vi "WSVCAP SHL Host TL Tester.vi"() -> ()   [LabVIEW 2012]
uses:
  Type Defs/WSVCAP SHL DUT Number Enum.ctl
  <vilib>/userdefined/High Color/nirio_resource_hc.ctl
  Type Defs/WSVCAP SHL Tester System Cluster.ctl
  Type Defs/WSVCAP SHL I2C DUT Mask Mode Enum.ctl
panel:
  in  "C3 Cap DAC":u8=144 caption="B Data In" format="0x%02x"
  in  "C2 Cap DAC":u8=144 caption="B Data In" format="0x%02x"
  in  "C1 Cap DAC":u8=144 caption="B Data In" format="0x%02x"
  in  "Set Cap DAC":bool
  in  "CP 35V":bool
  in  "CP 23.75V":bool
  in  "DVA On":bool
  in  "DVA Off":bool
  in  "CP 44V":bool
  in  "CP 40.25V":bool
  in  "Read Data DUT CMD":string caption="Read Data Out"
  in  "Read DUT":bool
  in  "CP On":bool
  in  "CP Off":bool
  in  "Write DUT":bool
  in  "Write Data DUT":string caption="Write Data Out"
  out "Read Data DUT Out":string caption="Data In"
  in  "Stop RFFE Cycle":bool
  in  "Start RFFE Cycle":bool
  in  "Command":string[](array[string])=["702013B3B3B", "70201000000"]
  in  "Post CMd Delay":dbl[](array[numeric])=[1.2e-05, 5.4e-05] min=0.0 max=0.5 format="%#.0p s"
  in  "Number of Commands":u32=2 min=1 max=4 step=1
  out "Cycle Count":u64=2 min=1 max=4 step=1
  in  "Monitor":bool
  out "AD7747 Values":string[][](table)
  in  "Mode":enum32{"C1", "C2", "C3", "All", "Single"}(radio)
  in  "RFFE Slave Address":u8=144 caption="Slave Address" format="0x%02x"
  out "Activity Log":string
  out "Simulate FPGA":bool
  out "Online":bool
  out "FPGA Resource":T1
  out "Status":string
  out "Busy":bool
  in  "I2C Bytes to Read":u8=1 caption="Bytes" min=1 max=4 step=1
  in  "Device":enum32{"C1", "C2", "C3"}(radio)
  in  "Exit":bool
  out "Read Data I2C":u8[](array[numeric]) caption="Data In" format="0x%02x"
  in  "Read Reg I2C":u8 caption="Register" format="0x%02x"
  in  "Read I2C":bool
  in  "DUT":T2
  in  "Write Data I2C":u8 caption="Data Out" format="0x%02x"
  in  "Write Reg I2C":u8=144 caption="Register" format="0x%02x"
  in  "I2C Init":bool
  in  "Init Data":u8[](array[numeric])=[164, 160, 14, 33] caption="Data Out" format="0x%02x"
  in  "Init Reg":u8[](array[numeric])=[191, 7, 9, 10] caption="Register" format="0x%02x"
  in  "Write I2C":bool
  in  "I2C Slave Address":u8=144 caption="Slave Address" format="0x%02x"
  in  "RFFE Clock Rate (Hz)":dbl=1000000.0 caption="Clock Rate" format="%.1p Hz"
  in  "I2C Clock Rate (Hz)":dbl=100000.0 caption="Clock Rate" format="%.0p Hz"
  in  "Error":errorcluster
  # "WS1050 Tester"
  # "AD7747 (I2C)"
  # "C1"
  # "C2"
  # "C3"
  # "DUT Control (RFFE)"
  # "DUT Cycling (RFFE)"
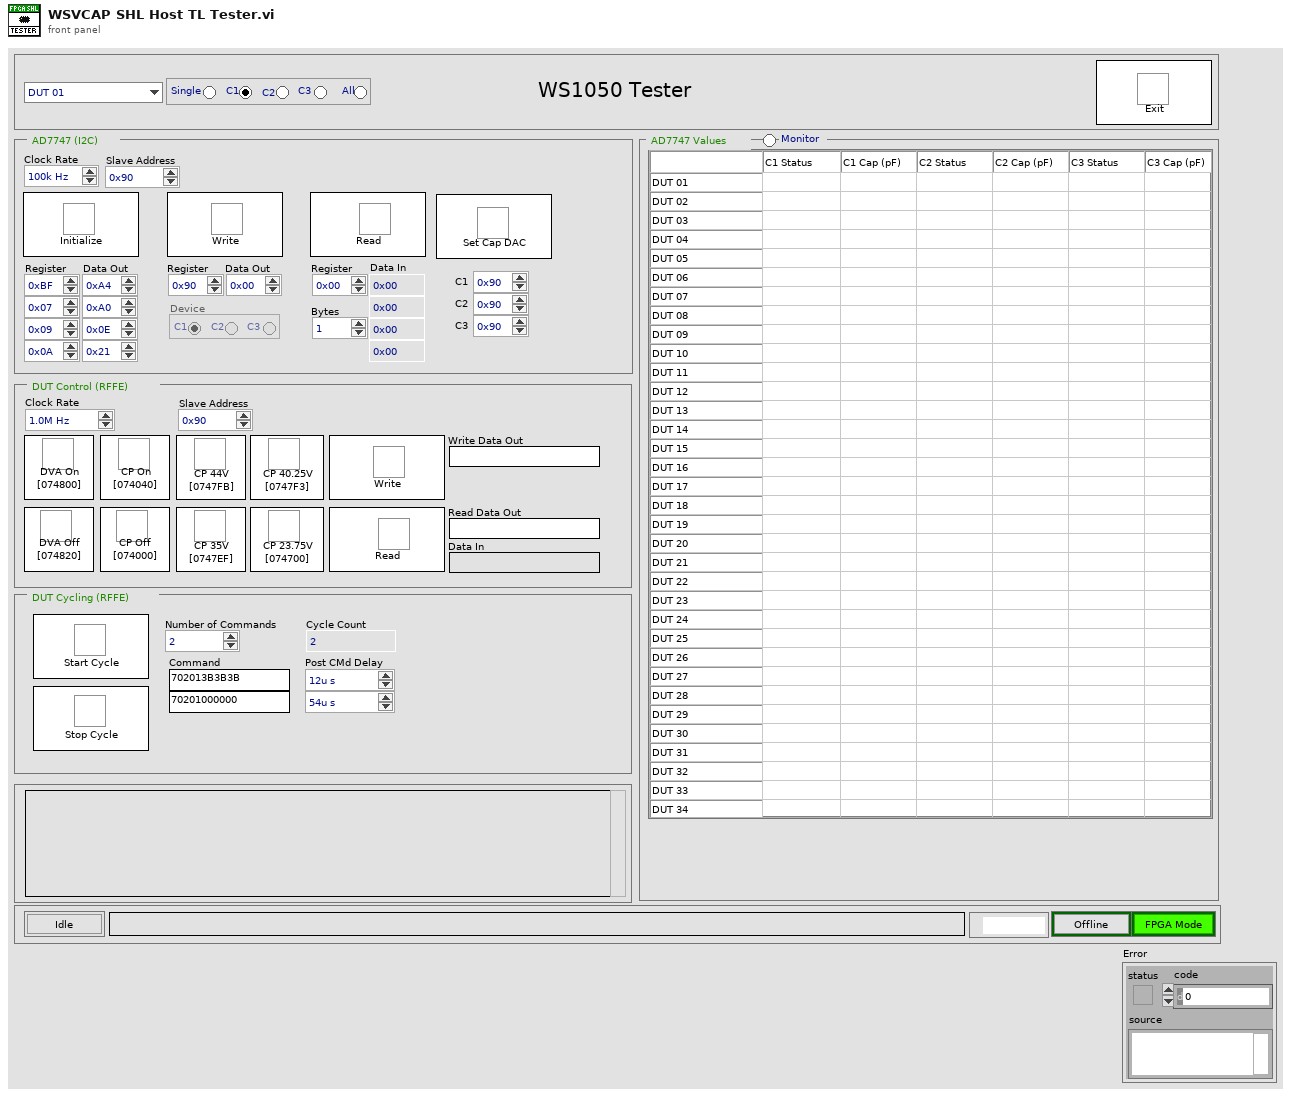
[diagram p1: front panel]
types:
  T1 = typedef "nirio_resource_hc.ctl" = tag
  T2 = typedef "WSVCAP SHL DUT Number Enum.ctl" = enum16{"DUT 01", "DUT 02", "DUT 03", "DUT 04", "DUT 05", "DUT 06", "DUT 07", "DUT 08", "DUT 09", "DUT 10", "DUT 11", "DUT 12", "DUT 13", "DUT 14", "DUT 15", "DUT 16", "DUT 17", "DUT 18", "DUT 19", "DUT 20", "DUT 21", "DUT 22", "DUT 23", "DUT 24", "DUT 25", "DUT 26", "DUT 27", "DUT 28", "DUT 29", "DUT 30", "DUT 31", "DUT 32", "DUT 33", "DUT 34", "DUT 35", "DUT 36"}
  T3 = typedef "WSVCAP SHL Tester System Cluster.ctl" = cluster{"I2C Monitor":bool, "SPI Cyle":bool, "SPI Mode":enum32{"Write/Read", "Cycle"}, "RFFE Cyle":bool, "RFFE Mode":enum32{"Write/Read", "Cycle"}}
  T4 = typedef "WSVCAP SHL Core System Cluster.ctl" = cluster{"Settings":T5, "FPGA Resource":tag, "Online":bool, "I2C Wait Ticks":u32, "SPI Wait Ticks":u32, "RFFE Wait Ticks":u32}
  T5 = typedef "WSVCAP SHL I2C Settings Cluster.ctl" = cluster{"FPGA Resource Name":string, "I2C Slave Address":u8, "I2C Clock Rate (Hz)":dbl, "SPI Clock Rate (Hz)":dbl, "RFFE Slave Address":u8, "RFFE Clock Rate (Hz)":dbl, "Simulate FPGA":bool, "C1 Cap DAC Default":u8, "C2 Cap DAC Default":u8, "C3 Cap DAC Default":u8}
  T6 = enum8{"Enabled", "Disabled", "Disabled and Grayed Out"}
  T7 = typedef "WSVCAP SHL I2C DUT Mask Mode Enum.ctl" = enum16{"Custom", "C1", "C2", "C3", "All"}
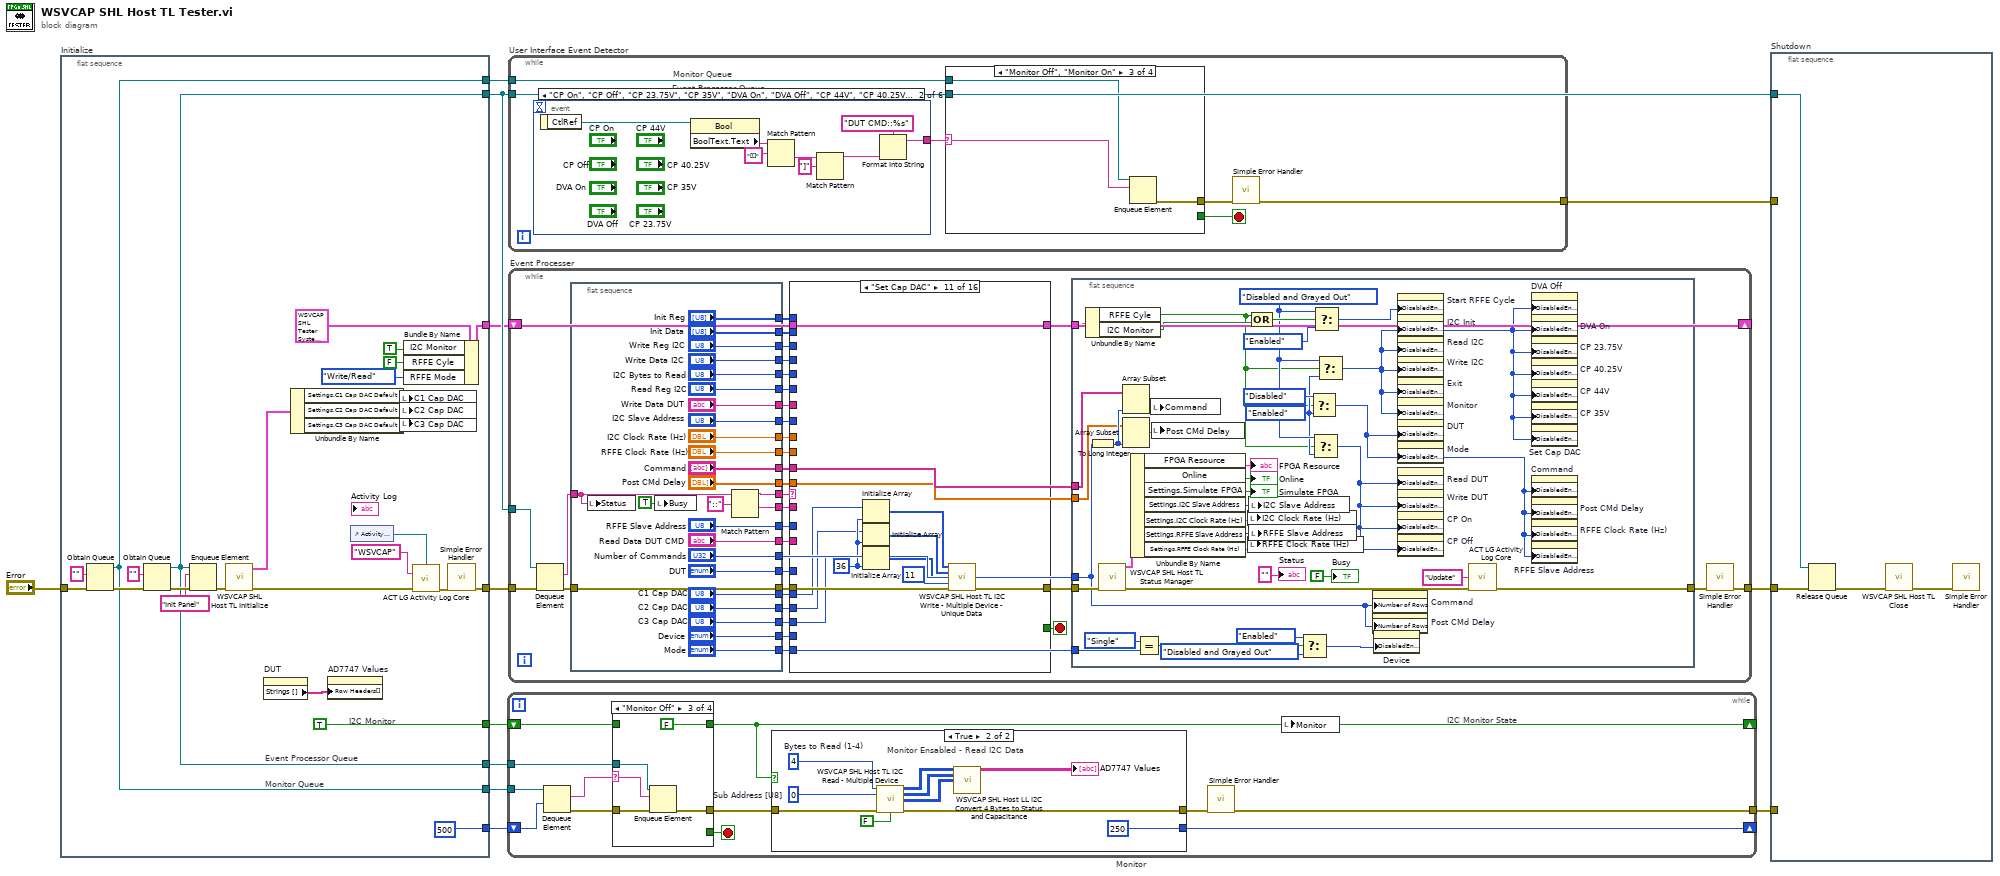
[diagram p0: block diagram]
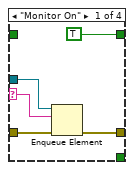
[diagram p2: hidden frame]
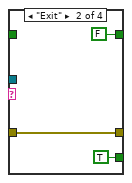
[diagram p3: hidden frame]
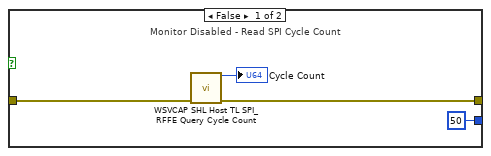
[diagram p5: hidden frame]
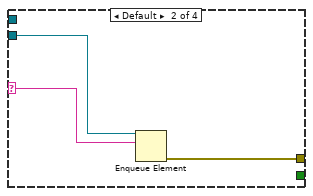
[diagram p7: hidden frame]
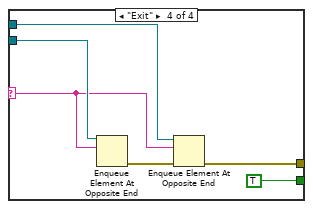
[diagram p8: hidden frame]
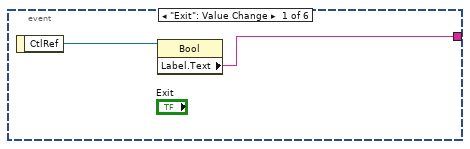
[diagram p9: hidden frame]
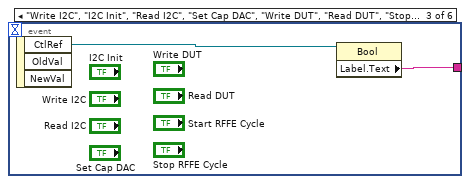
[diagram p10: hidden frame]
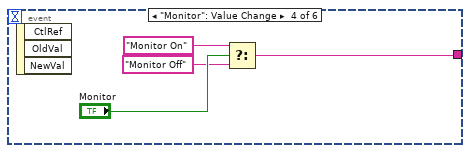
[diagram p11: hidden frame]
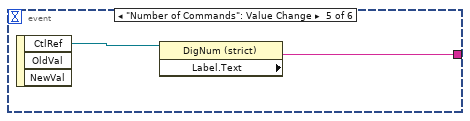
[diagram p12: hidden frame]
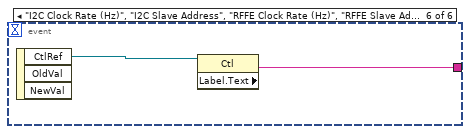
[diagram p13: hidden frame]
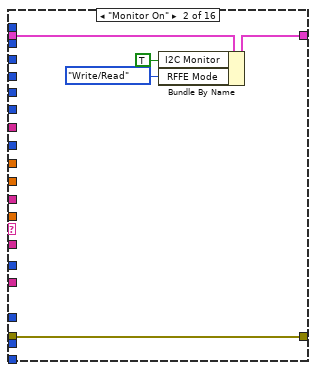
[diagram p15: hidden frame]
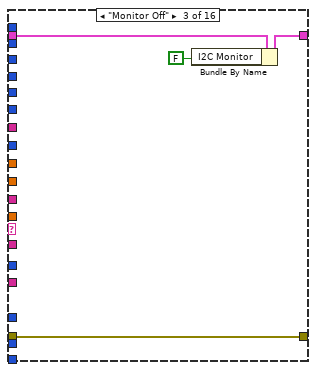
[diagram p16: hidden frame]
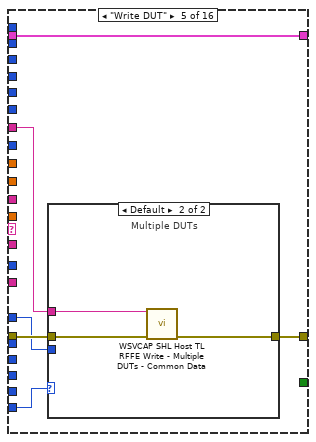
[diagram p18: hidden frame]
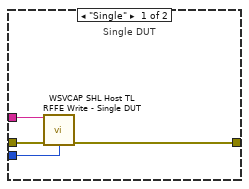
[diagram p19: hidden frame]
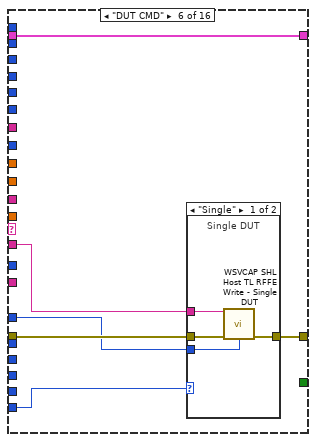
[diagram p20: hidden frame]
diagram:
  n1 = flat-sequence "Initialize" {
    tunnel: "Error" -> [w29]
    tunnel: [w27] -> w11
    tunnel: [TRUE ("Monitor")] -> w2
    tunnel: [w34] -> w7
    tunnel: [w25] -> w6
    tunnel: [w22] -> w5
    tunnel: [w27] -> w4
    tunnel: [w22] -> w3
    tunnel: [500 ("Wait Time (500ms)")] -> w1
    frame #0 {
      # "I2C Monitor"
      # "Monitor Queue"
      # "Event Processor Queue"
      n2 = Obtain Queue(element data type="" ("name (unnamed)"), error in (no error)=w29) -> (queue out=w22:refnum<queue>, error out=w28:errorcluster)  [unwired: 3 in, 1 out]
      n3 = Obtain Queue(element data type="" ("name (unnamed)"), error in (no error)=w28) -> (queue out=w27:refnum<queue>, error out=w37:errorcluster)  [unwired: 3 in, 1 out]
      n4 = Enqueue Element(queue=w27, element="Init Panel" ("name (unnamed)"), error in (no error)=w37) -> (error out=w19:errorcluster)  [unwired: 1 in, 2 out]
      n5 = call "WSVCAP SHL Host TL Initialize.vi"("error in"=w19) -> ("System"=w17:T4, "error out"=w18:errorcluster)  [unwired: 13 in]
      n6 = property on="DUT" class="Enum (strict)"() -> ("Strings []"=w20:string[])  [unwired: 2 in, 2 out]
      n7 = Unbundle By Name(w17) -> ("Settings.C1 Cap DAC Default"=w16:u8, "Settings.C2 Cap DAC Default"=w15:u8, "Settings.C3 Cap DAC Default"=w14:u8)
      n8 = property on="AD7747 Values" class="Tbl (strict)"("Row Headers[]"=w20) -> ()  [unwired: 2 in, 2 out]
      n9 = control-ref of="Activity Log"() -> (w33:refnum<vi>)
      n10 = local write "C1 Cap DAC"(w16) -> ()
      n11 = local write "C2 Cap DAC"(w15) -> ()
      n12 = local write "C3 Cap DAC"(w14) -> ()
      n13 = Bundle By Name(cluster=T3 {"I2C Monitor"=TRUE, "SPI Cyle"=TRUE, "SPI Mode"=enum."Write/Read", "RFFE Cyle"=FALSE, "RFFE Mode"=enum."Write/Read"}, "I2C Monitor"=TRUE, "RFFE Cyle"=FALSE ("I2C Monitor"), "RFFE Mode"=enum32{"Write/Read", "Cycle"}."Write/Read" ("SPI Mode")) -> (w25:T3)
      n14 = call "ACT LG Activity Log Core.vi"("Display Ref"=w33, "Source"="WSVCAP", "Error In (no error)"=w18) -> ("Error Out"=w35:errorcluster)  [unwired: 11 in, 1 out]
      n15 = call <vilib>:"Simple Error Handler.vi"("error in (no error)"=w35) -> ("error out"=w34:errorcluster)  [unwired: 4 in, 4 out]
    }
  }
  n16 = while "Monitor" {
    tunnel: [w42] -> w8
    shift-right: [w41] -> _
    shift-left: w2 -> [w48]
    tunnel: w5 -> [w46]
    tunnel: w4 -> [w45]
    shift-right: [w40] -> _
    shift-left: w1 -> [w39]
    stop <- w43 stop-if-true
    # "I2C Monitor State"
    n17 = Dequeue Element(queue=w46, timeout in ms (-1)=w39) -> (element=w49:string, error out=w47:errorcluster)  [unwired: 1 in, 2 out]
    n18 = case shown="\"Monitor Off\"" w49 {
      selector: w49 -> [w52 _ w60 _]
      tunnel: [TRUE FALSE FALSE w65] -> w41
      tunnel: w48 -> [_ _ _ w65]
      tunnel: w47 -> [w54 w57 w62 w64]
      tunnel: [w53 w57 w61 w64] -> w44
      tunnel: w45 -> [w51 _ w59 _]
      tunnel: [_ TRUE _ _] -> w43
      frame "Monitor On" {
        n19 = Enqueue Element(queue=w51, element=w52, error in (no error)=w54) -> (error out=w53:errorcluster)  [unwired: 1 in, 2 out]
      }
      frame "Exit" {
      }
      frame "Monitor Off" {
        n20 = Enqueue Element(queue=w59, element=w60, error in (no error)=w62) -> (error out=w61:errorcluster)  [unwired: 1 in, 2 out]
      }
      frame Default {
      }
    }
    n21 = case shown="True" w41 {
      tunnel: [w67 w73] -> w50
      tunnel: w44 -> [w68 w74]
      tunnel: [50 ("Wait Time (500ms)") 250 ("Wait Time (500ms)")] -> w40
      frame False {
        # "Monitor Disabled - Read SPI Cycle Count"
        n22 = call "WSVCAP SHL Host TL SPI_RFFE Query Cycle Count.vi"("error in"=w68) -> ("Cycle Count"=→"Cycle Count":u64, "error out"=w67:errorcluster)  [unwired: 13 in]
      }
      frame True {
        w78 = u8 4  # Bytes to Read (1-4)
        w79 = u8 0  # Sub Address [U8]
        # "Monitor Ensabled - Read I2C Data"
        n23 = call "WSVCAP SHL Host TL I2C Read - Multiple Device.vi"("Bytes to Read (1-4)"=w78, "Sub Address [U8]"=w79, "error in"=w74, "Log (T)"=FALSE) -> ("C1:1-36 Read Data [U8]"=w77:u8[][], "C2:1-36 Read Data [U8]"=w76:u8[][], "C3:1-36 Read Data [U8]"=w72:u8[][], "error out"=w73:errorcluster)  [unwired: 8 in]
        n24 = call "WSVCAP SHL Host LL I2C Convert 4 Bytes to Status and Capacitance.vi"("C1:1-36 Read Data [U8]"=w77, "C2_1-36 Read Data [U8]"=w76, "C3_1-36 Read Data [U8]"=w72) -> ("AD7747 Values"=→"AD7747 Values":string[][])  [unwired: 12 in]
      }
    }
    n25 = call <vilib>:"Simple Error Handler.vi"("error in (no error)"=w50) -> ("error out"=w42:errorcluster)  [unwired: 4 in, 4 out]
    n26 = local write "Monitor"(w41) -> ()
  }
  n27 = while "User Interface Event Detector" {
    tunnel: w11 -> [w84]
    tunnel: [w81] -> w9
    tunnel: w3 -> [w80]
    stop <- w82 stop-if-true
    # "Monitor Queue"
    # "Event Processor Queue"
    n28 = event shown="[1] \"CP On\", \"CP Off\", \"CP 23.75V\", \"CP 35V\", \"DVA On\", \"DVA Off\", \"CP 44V\", \"CP 40.25V\": Value Change" {
      selector: _ -> [_ _ _ _ _ _]
      dyn-events: _ -> [_ _ _ _ _ _]
      timeout: _ -> [_ _ _ _ _ _]
      tunnel: [w98 w106 w109 w110 w115 w117] -> w85
      event "Exit": Value Change {
        n29 = event-data() -> ("CtlRef"=w99:refnum<vi>)  [unwired: 1 in]
        n30 = property class="Bool"(reference=w99) -> ("Label.Text"=w98:string)  [unwired: 1 in, 2 out]
      }
      event "CP On", "CP Off", "CP 23.75V", "CP 35V", "DVA On", "DVA Off", "CP 44V", "CP 40.25V": Value Change {
        n31 = event-data() -> ("CtlRef"=w107:refnum<vi>)  [unwired: 1 in]
        n32 = property class="Bool"(reference=w107) -> ("BoolText.Text"=w104:string)  [unwired: 1 in, 2 out]
        n33 = Match Pattern(string=w104, regular expression="[[]") -> (after substring=w102:string)  [unwired: 1 in, 3 out]
        n34 = Match Pattern(string=w102, regular expression="]") -> (before substring=w100:string)  [unwired: 1 in, 3 out]
        n35 = Format Into String(format string="DUT CMD::%s", w100) -> (resulting string=w106:string)  [unwired: 2 in, 1 out]
      }
      event "Write I2C", "I2C Init", "Read I2C", "Set Cap DAC", "Write DUT", "Read DUT", "Stop RFFE Cycle", "Start RFFE Cycle": Value Change {
        n36 = event-data() -> ("CtlRef"=w108:refnum<vi>)  [unwired: 1 in, 2 out]
        n37 = property class="Bool"(reference=w108) -> ("Label.Text"=w109:string)  [unwired: 1 in, 2 out]
      }
      event "Monitor": Value Change {
        n38 = event-data() -> ()  [unwired: 1 in, 3 out]
        n39 = Select(t="Monitor On" ("Label.Text"), s="Monitor", f="Monitor Off" ("Label.Text")) -> (s? t:f=w110:string)
      }
      event "Number of Commands": Value Change {
        n40 = event-data() -> ("CtlRef"=w114:refnum<vi>)  [unwired: 1 in, 2 out]
        n41 = property class="DigNum (strict)"(reference=w114) -> ("Label.Text"=w115:string)  [unwired: 1 in, 2 out]
      }
      event "I2C Clock Rate (Hz)", "I2C Slave Address", "RFFE Clock Rate (Hz)", "RFFE Slave Address", "Mode": Value Change {
        n42 = event-data() -> ("CtlRef"=w116:refnum<vi>)  [unwired: 1 in, 2 out]
        n43 = property class="Ctl"(reference=w116) -> ("Label.Text"=w117:string)  [unwired: 1 in, 2 out]
      }
    }
    n44 = case shown="\"Monitor Off\", \"Monitor On\"" w85 {
      selector: w85 -> [_ w88 w91 w92]
      tunnel: w84 -> [_ w87 _ w97]
      tunnel: [_ w86 w90 w94] -> w83
      tunnel: [_ _ _ TRUE] -> w82
      tunnel: w80 -> [_ _ w89 w93]
      frame "" {
      }
      frame Default {
        n45 = Enqueue Element(queue=w87, element=w88) -> (error out=w86:errorcluster)  [unwired: 2 in, 2 out]
      }
      frame "Monitor Off", "Monitor On" {
        n46 = Enqueue Element(queue=w89, element=w91) -> (error out=w90:errorcluster)  [unwired: 2 in, 2 out]
      }
      frame "Exit" {
        n47 = Enqueue Element At Opposite End(queue=w97, element=w92) -> (error out=w95:errorcluster)  [unwired: 2 in, 2 out]
        n48 = Enqueue Element At Opposite End(queue=w93, element=w92, error in (no error)=w95) -> (error out=w94:errorcluster)  [unwired: 1 in, 2 out]
      }
    }
    n49 = call <vilib>:"Simple Error Handler.vi"("error in (no error)"=w83) -> ("error out"=w81:errorcluster)  [unwired: 4 in, 4 out]
  }
  n50 = while "Event Processer" {
    tunnel: w11 -> [w151]
    tunnel: [w149] -> w10
    tunnel: w7 -> [w130]
    shift-right: [w125] -> _
    shift-left: w6 -> [w126]
    stop <- w150 stop-if-true
    n51 = Dequeue Element(queue=w151, error in (no error)=w130) -> (element=w147:string, error out=w145:errorcluster)  [unwired: 1 in, 2 out]
    n52 = flat-sequence {
      tunnel: ["I2C Clock Rate (Hz)"] -> w148
      tunnel: [w195] -> w146
      tunnel: w147 -> [w196]
      tunnel: [w215] -> w144
      tunnel: w145 -> [w215]
      tunnel: ["I2C Bytes to Read"] -> w143
      tunnel: ["I2C Slave Address"] -> w142
      tunnel: ["RFFE Clock Rate (Hz)"] -> w141
      tunnel: ["DUT"] -> w138
      tunnel: ["Init Data"] -> w137
      tunnel: ["Init Reg"] -> w136
      tunnel: ["Write Reg I2C"] -> w135
      tunnel: ["Write Data I2C"] -> w134
      tunnel: ["Read Reg I2C"] -> w133
      tunnel: ["Write Data DUT"] -> w132
      tunnel: ["Mode"] -> w122
      tunnel: ["Device"] -> w131
      tunnel: ["Command"] -> w128
      tunnel: ["Post CMd Delay"] -> w127
      tunnel: ["Number of Commands"] -> w129
      tunnel: ["RFFE Slave Address"] -> w124
      tunnel: ["Read Data DUT CMD"] -> w123
      tunnel: [w193] -> w121
      tunnel: ["C1 Cap DAC"] -> w120
      tunnel: ["C2 Cap DAC"] -> w119
      tunnel: ["C3 Cap DAC"] -> w118
      frame #0 {
        n53 = local write "Status"(w196) -> ()
        n54 = local write "Busy"(TRUE ("Busy")) -> ()
        n55 = Match Pattern(string=w196, regular expression="::") -> (before substring=w195:string, after substring=w193:string)  [unwired: 1 in, 2 out]
      }
    }
    n56 = case shown="\"Set Cap DAC\"" w146 {
      tunnel: w144 -> [w218 w223 w227 w229 w235 w248 w261 w285 w299 w307 w326 w340 w369 w371 w377 w382]
      tunnel: [w218 w223 w227 w229 w234 w247 w260 w284 w298 w306 w325 w339 w363 w371 w374 w380] -> w140
      tunnel: [_ _ _ _ _ _ _ _ _ _ _ _ _ TRUE _ _] -> w150
      tunnel: w148 -> [_ _ _ _ _ _ _ _ _ _ _ _ _ _ w376 _]
      tunnel: w143 -> [_ _ _ _ _ _ _ _ _ _ _ _ w365 _ _ _]
      tunnel: w142 -> [_ _ _ _ _ _ _ _ _ _ _ _ _ _ w375 _]
      tunnel: w141 -> [_ _ _ _ _ _ _ _ _ _ _ _ _ _ _ w381]
      tunnel: w138 -> [_ _ _ _ w232 w245 w258 w282 _ w304 _ w337 w368 _ _ _]
      tunnel: w137 -> [_ _ _ _ _ _ _ _ _ _ _ w334 _ _ _ _]
      tunnel: w136 -> [_ _ _ _ _ _ _ _ _ _ _ w335 _ _ _ _]
      tunnel: w135 -> [_ _ _ _ _ _ _ _ _ w302 _ _ _ _ _ _]
      tunnel: w134 -> [_ _ _ _ _ _ _ _ _ w301 _ _ _ _ _ _]
      tunnel: w133 -> [_ _ _ _ _ _ _ _ _ _ _ _ w366 _ _ _]
      tunnel: w132 -> [_ _ _ _ w231 _ _ _ _ _ _ _ _ _ _ _]
      tunnel: w122 -> [_ _ _ _ w233 w246 w259 w283 _ w305 _ w338 _ _ _ _]
      tunnel: w131 -> [_ _ _ _ _ _ _ _ _ w303 _ w336 w367 _ _ _]
      tunnel: w128 -> [_ _ _ _ _ _ _ w281 _ _ _ _ _ _ _ _]
      tunnel: w127 -> [_ _ _ _ _ _ _ w280 _ _ _ _ _ _ _ _]
      tunnel: [w217 w221 w225 w228 w230 w244 w257 w278 w295 w300 w332 w333 w362 w370 w373 w379] -> w125
      tunnel: w126 -> [w217 w222 w226 w228 w230 w244 w257 w279 w296 w300 w332 w333 w362 w370 w373 w379]
      tunnel: w124 -> [_ _ _ _ _ _ _ _ _ _ _ _ _ _ _ w378]
      tunnel: w123 -> [_ _ _ _ _ _ w256 _ _ _ _ _ _ _ _ _]
      tunnel: w121 -> [_ _ _ _ _ w243 _ _ _ _ _ _ _ _ _ _]
      tunnel: w120 -> [_ _ _ _ _ _ _ w276 _ _ w324 _ _ _ _ _]
      tunnel: w119 -> [_ _ _ _ _ _ _ w275 _ _ w323 _ _ _ _ _]
      tunnel: w118 -> [_ _ _ _ _ _ _ w274 _ _ w322 _ _ _ _ _]
      frame Default {
      }
      frame "Monitor On" {
        n57 = Bundle By Name(cluster=w222, "I2C Monitor"=TRUE, "RFFE Mode"=enum32{"Write/Read", "Cycle"}."Write/Read" ("SPI Mode")) -> (w221:T3)
      }
      frame "Monitor Off" {
        n58 = Bundle By Name(cluster=w226, "I2C Monitor"=FALSE) -> (w225:T3)
      }
      frame "Number of Commands" {
      }
      frame "Write DUT" {
        n59 = case shown="Default" w233 {
          tunnel: w235 -> [w239 w242]
          tunnel: [w236 w241] -> w234
          tunnel: w232 -> [w237 _]
          tunnel: w231 -> [w238 w240]
          frame "Single" {
            # "Single DUT"
            n60 = call "WSVCAP SHL Host TL RFFE Write - Single DUT.vi"("Data Out"=w238, "error in"=w239, "DUT"=w237) -> ("error out"=w236:errorcluster)  [unwired: 12 in]
          }
          frame Default {
            # "Multiple DUTs"
            n61 = call "WSVCAP SHL Host TL RFFE Write - Multiple DUTs - Common Data.vi"("Data Out"=w240, "error in"=w242) -> ("error out"=w241:errorcluster)  [unwired: 13 in]
          }
        }
      }
      frame "DUT CMD" {
        n62 = case shown="\"Single\"" w246 {
          tunnel: w248 -> [w252 w255]
          tunnel: [w249 w254] -> w247
          tunnel: w245 -> [w250 _]
          tunnel: w243 -> [w251 w253]
          frame "Single" {
            # "Single DUT"
            n63 = call "WSVCAP SHL Host TL RFFE Write - Single DUT.vi"("Data Out"=w251, "error in"=w252, "DUT"=w250) -> ("error out"=w249:errorcluster)  [unwired: 12 in]
          }
          frame Default {
            # "Multiple DUTs"
            n64 = call "WSVCAP SHL Host TL RFFE Write - Multiple DUTs - Common Data.vi"("Data Out"=w253, "error in"=w255) -> ("error out"=w254:errorcluster)  [unwired: 13 in]
          }
        }
      }
      frame "Read DUT" {
        n65 = case shown="\"Single\"" w259 {
          tunnel: w261 -> [w266 w273]
          tunnel: [w264 w272] -> w260
          tunnel: w258 -> [w265 w269]
          tunnel: w256 -> [w262 w271]
          frame "Single" {
            # "Single DUT"
            n66 = call "WSVCAP SHL Host TL RFFE Read - Single DUT.vi"("Data Out"=w262, "error in"=w266, "DUT"=w265) -> ("Data In"=→"Read Data DUT Out":string, "error out"=w264:errorcluster)  [unwired: 11 in]
          }
          frame Default {
            # "Multiple DUTs"
            n67 = To Long Integer(number=w269) -> (32bit integer=w268:i32)
            n68 = call "WSVCAP SHL Host TL RFFE Read - Multiple DUTs - Common Data.vi"("Data Out"=w271, "error in"=w273) -> ("RFFE Data In"=w270:string[], "error out"=w272:errorcluster)  [unwired: 12 in]
            n69 = Index Array(array=w270, index=w268) -> (element=w267:string)
            n70 = local write "Read Data DUT Out"(w267) -> ()
          }
        }
      }
      frame "Start RFFE Cycle" {
        n71 = case shown="Default" w283 {
          tunnel: w285 -> [w290 w294]
          tunnel: [w289 w293] -> w284
          tunnel: w282 -> [w288 _]
          tunnel: w281 -> [w287 w292]
          tunnel: w280 -> [w286 w291]
          tunnel: w276 -> [_ _]
          tunnel: w275 -> [_ _]
          tunnel: w274 -> [_ _]
          frame Default {
            # "Single DUT"
            n72 = call "WSVCAP SHL Host TL RFFE Write Cycle - Single DUT.vi"("Data Out (Cycle Commands)"=w287, "Post Command Delay"=w286, "error in"=w290, "DUT"=w288) -> ("error out"=w289:errorcluster)  [unwired: 11 in]
          }
          frame "All" {
            # "Multiple DUTs"
            n73 = call "WSVCAP SHL Host TL RFFE Write Cycle - Multiple DUTs - Common Data.vi"("Data Out (Cycle Commands)"=w292, "Post Command Delay"=w291, "error in"=w294) -> ("error out"=w293:errorcluster)  [unwired: 12 in]
          }
        }
        n74 = Bundle By Name(cluster=w279, "RFFE Cyle"=TRUE ("SPI Cyle")) -> (w278:T3)
      }
      frame "Stop RFFE Cycle" {
        n75 = call "WSVCAP SHL Host TL RFFE Stop Write Cycle.vi"("error in"=w299) -> ("error out"=w298:errorcluster)  [unwired: 14 in]
        n76 = Bundle By Name(cluster=w296, "RFFE Cyle"=FALSE ("SPI Cyle")) -> (w295:T3)
      }
      frame "Write I2C" {
        n77 = case shown="\"Single\"" w305 {
          selector: w305 -> [_ w317]
          tunnel: w307 -> [w313 w321]
          tunnel: [w312 w320] -> w306
          tunnel: w304 -> [w310 _]
          tunnel: w302 -> [w309 w319]
          tunnel: w303 -> [w311 _]
          tunnel: w301 -> [w308 w318]
          frame "Single" {
            # "Single DUT"
            n78 = call "WSVCAP SHL Host TL I2C Write - Single Device.vi"("Sub Address [U8]"=w309, "Data Out [U8]"=w308, "error in"=w313, "DUT"=w310, "Device"=w311) -> ("error out"=w312:errorcluster)  [unwired: 10 in]
          }
          frame Default {
            # "Multiple DUTs"
            n79 = Format Into String(w317) -> (resulting string=w316:string)  [unwired: 3 in, 1 out]
            n80 = Scan From String(input string=w316, default 1=WSVCAP_SHL_I2C_DUT_Mask_Mode_Enum."All" ("DUT Mask Mode (All)")) -> (output 1=w314:T7)  [unwired: 3 in, 3 out]
            n81 = call "WSVCAP SHL Host TL I2C Write - Multiple Device - Common Data.vi"("Sub Address"=w319, "Data Out [U8]"=w318, "error in"=w321, "DUT Mask Mode (All)"=w314) -> ("error out"=w320:errorcluster)  [unwired: 11 in]
          }
        }
      }
      frame "Set Cap DAC" {
        w331 = 36 ("dimension size")
        n82 = Initialize Array(w324, w331) -> (w330:u8[])
        n83 = Initialize Array(w323, w331) -> (w329:u8[])
        n84 = Initialize Array(w322, w331) -> (w328:u8[])
        n85 = call "WSVCAP SHL Host TL I2C Write - Multiple Device - Unique Data.vi"("C1 Data"=w330, "C2 Data"=w329, "C3 Data"=w328, "Sub Address"=u8 11, "error in"=w326) -> ("error out"=w325:errorcluster)  [unwired: 10 in]
      }
      frame "I2C Init" {
        n86 = for {
          tunnel: w338 -> [w345]
          tunnel: w337 -> [w344]
          tunnel: w336 -> [w343]
          tunnel: w335 -> [w342] mode=indexing
          tunnel: w334 -> [w341] mode=indexing
          shift-right: [w346] -> w339
          shift-left: w340 -> [w347]
          n87 = case shown="\"Single\"" w345 {
            selector: w345 -> [_ w355]
            tunnel: w347 -> [w353 w361]
            tunnel: [w352 w360] -> w346
            tunnel: w344 -> [w350 _]
            tunnel: w343 -> [w351 _]
            tunnel: w342 -> [w349 w359]
            tunnel: w341 -> [w348 w358]
            frame "Single" {
              # "Single DUT"
              n88 = call "WSVCAP SHL Host TL I2C Write - Single Device.vi"("Sub Address [U8]"=w349, "Data Out [U8]"=w348, "error in"=w353, "DUT"=w350, "Device"=w351) -> ("error out"=w352:errorcluster)  [unwired: 10 in]
            }
            frame Default {
              # "Multiple DUTs"
              n89 = Format Into String(w355) -> (resulting string=w357:string)  [unwired: 3 in, 1 out]
              n90 = Scan From String(input string=w357, default 1=WSVCAP_SHL_I2C_DUT_Mask_Mode_Enum."All" ("DUT Mask Mode (All)")) -> (output 1=w354:T7)  [unwired: 3 in, 3 out]
              n91 = call "WSVCAP SHL Host TL I2C Write - Multiple Device - Common Data.vi"("Sub Address"=w359, "Data Out [U8]"=w358, "error in"=w361, "DUT Mask Mode (All)"=w354) -> ("error out"=w360:errorcluster)  [unwired: 11 in]
            }
          }
        }
      }
      frame "Read I2C" {
        n92 = call "WSVCAP SHL Host TL I2C Read - Single Device.vi"("Bytes to Read (1-4)"=w365, "Sub Address [U8]"=w366, "error in"=w369, "DUT"=w368, "Device"=w367) -> ("Device Data"=→"Read Data I2C":u8[], "error out"=w363:errorcluster)  [unwired: 9 in]
      }
      frame "Exit" {
      }
      frame "I2C Clock Rate (Hz)", "I2C Slave Address" {
        n93 = call "WSVCAP SHL Host TL I2C Configure.vi"("I2C_Slave Address"=w375, "Clock Rate (Hz)"=w376, "error in"=w377) -> ("error out"=w374:errorcluster)  [unwired: 11 in, 1 out]
      }
      frame "RFFE Clock Rate (Hz)", "RFFE Slave Address" {
        n94 = call "WSVCAP SHL Host TL RFFE Configure.vi"("RFFE Slave Address"=w378, "Clock Rate (Hz)"=w381, "error in"=w382) -> ("error out"=w380:errorcluster)  [unwired: 11 in, 1 out]
      }
    }
    n95 = flat-sequence {
      tunnel: [w177] -> w139
      tunnel: w140 -> [w187]
      tunnel: w129 -> [w176]
      tunnel: w128 -> [w174]
      tunnel: w127 -> [w172]
      tunnel: w125 -> [w170]
      tunnel: w122 -> [w160]
      frame #0 {
        w164 = T6."Enabled" ("Disabled")
        w165 = T6."Disabled and Grayed Out" ("Disabled")
        n96 = Unbundle By Name(w170) -> ("RFFE Cyle"=w163:bool, "I2C Monitor"=w169:bool)
        n97 = To Long Integer(number=w176) -> (32bit integer=w175:i32)
        n98 = call "WSVCAP SHL Host TL Status Manager.vi"("error in"=w187) -> ("System Out"=w186:T4, "error out"=w179:errorcluster)  [unwired: 13 in]
        n99 = Array Subset(array=w174, length=w175) -> (w173:string[])  [unwired: 1 in]
        n100 = Array Subset(array=w172, length=w175) -> (w171:dbl[])  [unwired: 1 in]
        n101 = Unbundle By Name(w186) -> ("FPGA Resource"=→"FPGA Resource":tag, "Online"=→"Online":bool, "Settings.Simulate FPGA"=→"Simulate FPGA":bool, "Settings.I2C Slave Address"=w185:u8, "Settings.I2C Clock Rate (Hz)"=w184:dbl, "Settings.RFFE Slave Address"=w161:u8, "Settings.RFFE Clock Rate (Hz)"=w183:dbl)
        n102 = Equal?(x=enum32{"C1", "C2", "C3", "All", "Single"}."Single" ("Mode"), y=w160) -> (x = y?=w156:bool)
        n103 = local write "Command"(w173) -> ()
        n104 = local write "Post CMd Delay"(w171) -> ()
        n105 = local write "I2C Clock Rate (Hz)"(w184) -> ()
        n106 = local write "RFFE Clock Rate (Hz)"(w183) -> ()
        n107 = local write "I2C Slave Address"(w185) -> ()
        n108 = local write "RFFE Slave Address"(w161) -> ()
        n109 = Compound Arithmetic op=OR(w163, w169) -> (w166:bool)
        n110 = Select(t=T6."Enabled" ("Disabled"), s=w156, f=T6."Disabled and Grayed Out" ("Disabled")) -> (s? t:f=w155:T6)
        n111 = Select(t=T6."Disabled" ("Disabled"), s=w163, f=w164) -> (s? t:f=w154:T6)
        n112 = Select(t=w165, s=w163, f=w164) -> (s? t:f=w152:T6)
        n113 = Select(t=w165, s=w166, f=T6."Enabled" ("Disabled")) -> (s? t:f=w162:T6)
        n114 = Select(t=w165, s=w163, f=w164) -> (s? t:f=w153:T6)
        n115 = property on="Command" class="Arr (strict)"("Number of Rows"=w176) -> ()  [unwired: 2 in, 2 out]
        n116 = property on="Post CMd Delay" class="Arr (strict)"("Number of Rows"=w176) -> ()  [unwired: 2 in, 2 out]
        n117 = property on="Device" class="RadioBtnsControl (strict)"("DisabledEnum"=w155) -> ()  [unwired: 2 in, 2 out]
        n118 = property on="Start RFFE Cycle" class="Bool"("DisabledEnum"=w162) -> ()  [unwired: 2 in, 2 out]
        n119 = property on="I2C Init" class="Bool"("DisabledEnum"=w153) -> ()  [unwired: 2 in, 2 out]
        n120 = property on="Read I2C" class="Bool"("DisabledEnum"=w153) -> ()  [unwired: 2 in, 2 out]
        n121 = property on="Write I2C" class="Bool"("DisabledEnum"=w153) -> ()  [unwired: 2 in, 2 out]
        n122 = property on="Exit" class="Bool"("DisabledEnum"=w153) -> ()  [unwired: 2 in, 2 out]
        n123 = property on="Monitor" class="Bool (strict)"("DisabledEnum"=w153) -> ()  [unwired: 2 in, 2 out]
        n124 = property on="DUT" class="Enum (strict)"("DisabledEnum"=w154) -> ()  [unwired: 2 in, 2 out]
        n125 = property on="Mode" class="RadioBtnsControl (strict)"("DisabledEnum"=w154) -> ()  [unwired: 2 in, 2 out]
        n126 = property on="Read DUT" class="Bool"("DisabledEnum"=w152) -> ()  [unwired: 2 in, 2 out]
        n127 = property on="Write DUT" class="Bool"("DisabledEnum"=w152) -> ()  [unwired: 2 in, 2 out]
        n128 = property on="CP On" class="Bool"("DisabledEnum"=w152) -> ()  [unwired: 2 in, 2 out]
        n129 = property on="CP Off" class="Bool"("DisabledEnum"=w152) -> ()  [unwired: 2 in, 2 out]
        n130 = call "ACT LG Activity Log Core.vi"("Log Line"="Update", "Error In (no error)"=w179) -> ("Error Out"=w177:errorcluster)  [unwired: 12 in, 1 out]
        n131 = property on="DVA Off" class="Bool"("DisabledEnum"=w153) -> ()  [unwired: 2 in, 2 out]
        n132 = property on="DVA On" class="Bool"("DisabledEnum"=w153) -> ()  [unwired: 2 in, 2 out]
        n133 = property on="CP 23.75V" class="Bool"("DisabledEnum"=w153) -> ()  [unwired: 2 in, 2 out]
        n134 = property on="CP 40.25V" class="Bool"("DisabledEnum"=w153) -> ()  [unwired: 2 in, 2 out]
        n135 = property on="CP 44V" class="Bool"("DisabledEnum"=w153) -> ()  [unwired: 2 in, 2 out]
        n136 = property on="CP 35V" class="Bool"("DisabledEnum"=w153) -> ()  [unwired: 2 in, 2 out]
        n137 = property on="Set Cap DAC" class="Bool"("DisabledEnum"=w153) -> ()  [unwired: 2 in, 2 out]
        n138 = property on="Command" class="Arr (strict)"("DisabledEnum"=w154) -> ()  [unwired: 2 in, 2 out]
        n139 = property on="Post CMd Delay" class="Arr (strict)"("DisabledEnum"=w154) -> ()  [unwired: 2 in, 2 out]
        n140 = property on="RFFE Clock Rate (Hz)" class="DigNum (strict)"("DisabledEnum"=w154) -> ()  [unwired: 2 in, 2 out]
        n141 = property on="RFFE Slave Address" class="DigNum (strict)"("DisabledEnum"=w154) -> ()  [unwired: 2 in, 2 out]
        "Busy" <- FALSE ("Busy")
        "Status" <- "" ("Status")
      }
    }
    n142 = call <vilib>:"Simple Error Handler.vi"("error in (no error)"=w139) -> ("error out"=w149:errorcluster)  [unwired: 4 in, 4 out]
  }
  n143 = flat-sequence "Shutdown" {
    tunnel: w11 -> [w386]
    tunnel: w10 -> [w385]
    tunnel: w9 -> [_]
    tunnel: w8 -> [_]
    frame #0 {
      n144 = Release Queue(queue=w386, error in (no error)=w385) -> (error out=w384:errorcluster)  [unwired: 1 in, 2 out]
      n145 = call "WSVCAP SHL Host TL Close.vi"("error in"=w384) -> ("error out"=w383:errorcluster)  [unwired: 14 in]
      n146 = call <vilib>:"Simple Error Handler.vi"("error in (no error)"=w383) -> ()  [unwired: 4 in, 5 out]
    }
  }
